vi "Create Sweeping Point Array.vi"(0 "Origin Point":T1 {"Latitude" format="%#_10g"; "Longitude" format="%#_10g"}, 5 "Image Width (m)":dbl, 7 "Diameter of polygon (km)":dbl, 9 "Bearing of first two points":dbl, 11 "Error In":errorcluster) -> (4 "Frame Points":T1[](array[typedef]) {"Latitude" format="%#_10g"; "Longitude" format="%#_10g"}, 6 "Bottom RIght corner":T1 {"Latitude" format="%#_10g"; "Longitude" format="%#_10g"}, 15 "Error Out":errorcluster)   [LabVIEW 2014]
uses:
  Lat Long Conversion/Controls/PointLatLon.ctl
  Lat Long Conversion/Decrement Bearing.vi
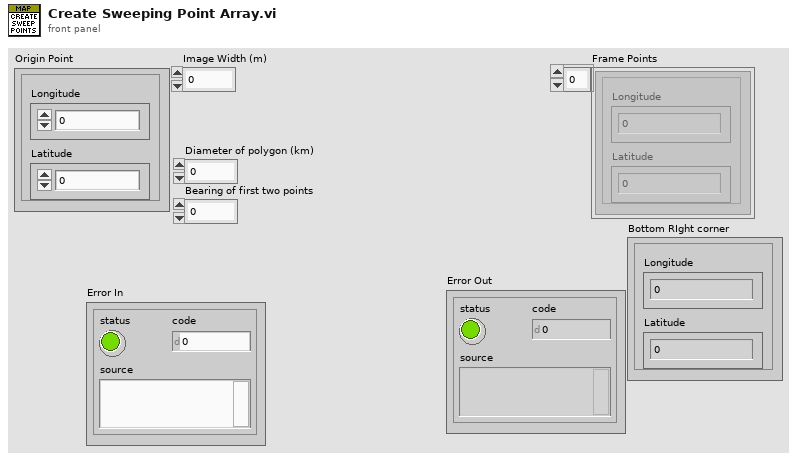
[diagram p1: front panel]
types:
  T1 = typedef "PointLatLon.ctl" = cluster{"Longitude":dbl, "Latitude":dbl}
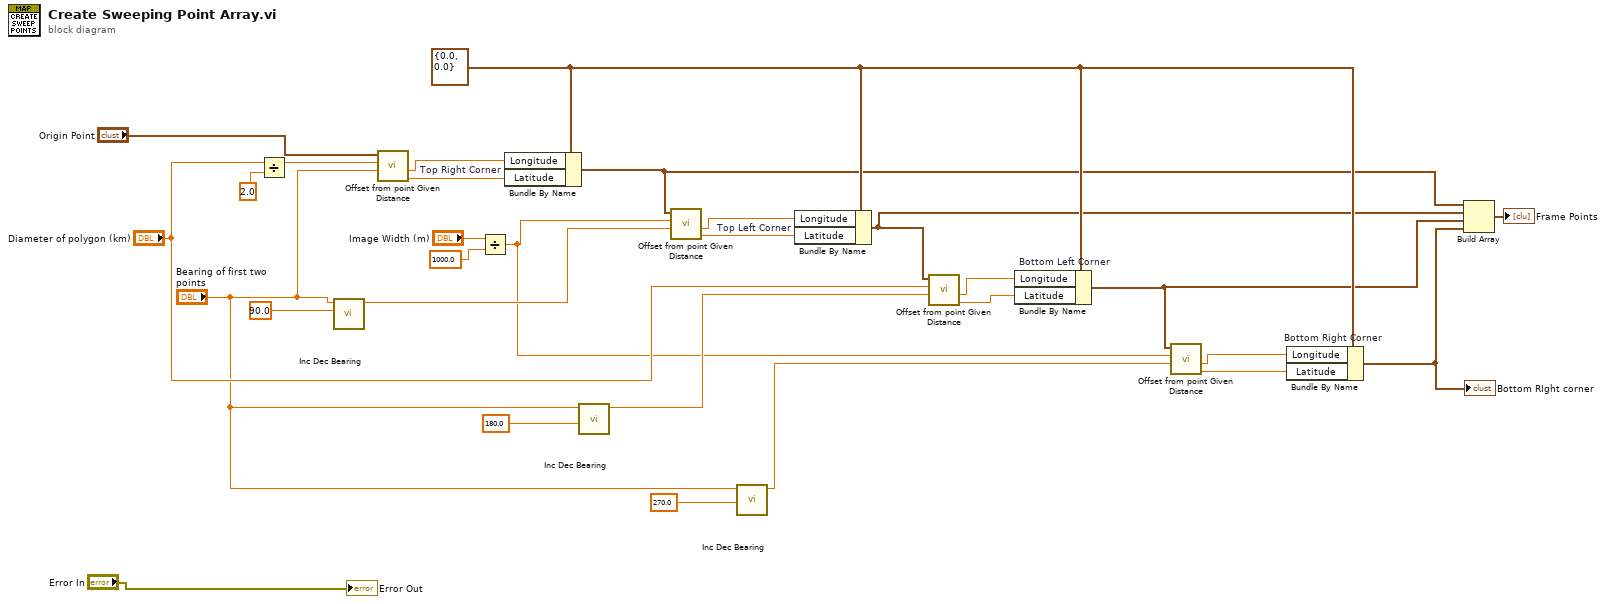
[diagram p0: block diagram]
diagram:
  w29 = T1 {"Longitude"=0.0, "Latitude"=0.0} ("Origin Point")
  n1 = Divide(x="Diameter of polygon (km)", y=2.0) -> (x/y=w24:dbl)
  n2 = call-poly "Inc Dec Bearing.vi"("Decrement Value"=90.0, "Bearing"="Bearing of first two points") -> ("New Bearing"=w17:dbl)  [unwired: 8 in, 1 out]
  n3 = call "Offset from point Given Distance.vi"("Bearing (clockwise from North)"="Bearing of first two points", "Distance (km)"=w24, "Origin Point"="Origin Point") -> ("Lat of new point"=w22:dbl, "Lon of new point"=w23:dbl)  [unwired: 5 in, 2 out]
  n4 = Divide(x="Image Width (m)", y=1000.0) -> (x/y=w7:dbl)
  n5 = Bundle By Name "Top Right Corner"(cluster=w29, "Longitude"=w23, "Latitude"=w22) -> (w21:T1)
  n6 = call-poly "Inc Dec Bearing.vi"("Decrement Value"=180.0, "Bearing"="Bearing of first two points") -> ("New Bearing"=w11:dbl)  [unwired: 8 in, 1 out]
  n7 = call "Offset from point Given Distance.vi"("Bearing (clockwise from North)"=w17, "Distance (km)"=w7, "Origin Point"=w21) -> ("Lat of new point"=w15:dbl, "Lon of new point"=w16:dbl)  [unwired: 5 in, 2 out]
  n8 = call-poly "Inc Dec Bearing.vi"("Decrement Value"=270.0, "Bearing"="Bearing of first two points") -> ("New Bearing"=w4:dbl)  [unwired: 8 in, 1 out]
  n9 = Bundle By Name "Top Left Corner"(cluster=w29, "Longitude"=w16, "Latitude"=w15) -> (w14:T1)
  n10 = call "Offset from point Given Distance.vi"("Bearing (clockwise from North)"=w11, "Distance (km)"="Diameter of polygon (km)", "Origin Point"=w14) -> ("Lat of new point"=w9:dbl, "Lon of new point"=w10:dbl)  [unwired: 5 in, 2 out]
  n11 = Bundle By Name "Bottom Left Corner"(cluster=w29, "Longitude"=w10, "Latitude"=w9) -> (w8:T1)
  n12 = call "Offset from point Given Distance.vi"("Bearing (clockwise from North)"=w4, "Distance (km)"=w7, "Origin Point"=w8) -> ("Lat of new point"=w2:dbl, "Lon of new point"=w3:dbl)  [unwired: 5 in, 2 out]
  n13 = Bundle By Name "Bottom Right Corner"(cluster=w29, "Longitude"=w3, "Latitude"=w2) -> (w28:T1)
  "Bottom RIght corner" <- w28
  n14 = Build Array(w21, w14, w8, w28) -> (→"Frame Points":T1[])
  "Error Out" <- "Error In"
